vi "Canny Edge Detection Image.vi"() -> ()   [LabVIEW 2018]
doc: "Canny Edge Detection Image: This example is a Canny edge detection example, which is an image processing system that utilizes the Canny edge detection algorithm. Canny edge detection is a classic edge detection algorithm aimed at discovering strong edges in images and minimizing false detections and false edges as much as possible。"
uses:
  vi.lib/VIRobotics/opencv_yiku/Mat/Mat_8U/Mat_8U.lvclass
  D:/Program Files/Company/National Instruments/LabVIEW 2018(64bit)/vi.lib/addons/VIRobotics/opencv_yiku/Mat/Mat/Mat.lvclass
  vi.lib/VIRobotics/opencv_yiku/Mat/Create_Mat_8U.vi
  vi.lib/VIRobotics/opencv_yiku/opencv_yiku.lvlib
panel:
  out "edge":picture
  # "Overview: Demonstrates how to find edges with Canny Edge Detection\nRequirements: Windows.\nInstructions: \n1.Run the VI"
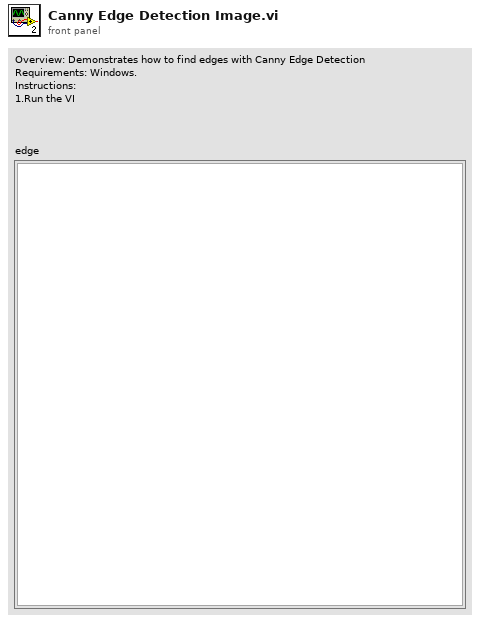
[diagram p1: front panel]
types:
  T1 = enum32{"COLOR_BGR2BGRA", "COLOR_BGRA2BGR", "COLOR_BGR2RGBA", "COLOR_RGBA2BGR", "COLOR_BGR2RGB", "COLOR_BGRA2RGBA", "COLOR_BGR2GRAY", "COLOR_RGB2GRAY", "COLOR_GRAY2BGR", "COLOR_GRAY2BGRA"}
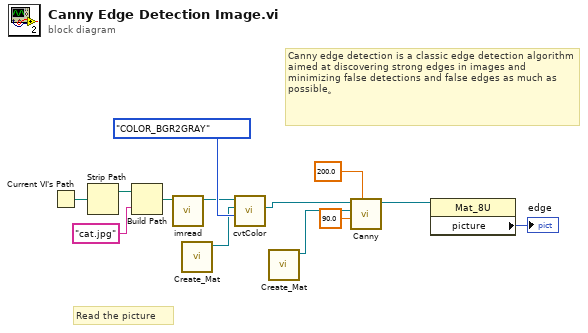
[diagram p0: block diagram]
diagram:
  # "Canny edge detection is a classic edge detection algorithm aimed at discovering strong edges in images and minimizing false detections and false edges as much as possible。"
  # "Read the picture"
  n1 = Current VI's Path() -> (path=w12:path)
  n2 = Strip Path(path=w12) -> (stripped path=w13:path)  [unwired: 1 out]
  n3 = Build Path(base path=w13, name or relative path="cat.jpg") -> (appended path=w10:path)
  n4 = call "imread.vi"("path"=w10) -> ("Mat out"=w8:refnum<class "Mat_8U.lvclass">)  [unwired: 9 in, 1 out]
  n5 = call-poly "Create_Mat.vi"() -> ("Mat_8U_out"=w2:refnum<class "Mat_8U.lvclass">)  [unwired: 10 in, 1 out]
  n6 = call "cvtColor.vi"("dstCn"=T1."COLOR_BGR2GRAY", "dst"=w2, "src"=w8) -> ("dst out"=w1:refnum<class "Mat_8U.lvclass">)  [unwired: 6 in, 2 out]
  n7 = call-poly "Create_Mat.vi"() -> ("Mat_8U_out"=w7:refnum<class "Mat_8U.lvclass">)  [unwired: 10 in, 1 out]
  n8 = call "Canny.vi"("threshold2"=200.0, "threshold1"=90.0, "dst in"=w7, "Mat in"=w1) -> ("dst out"=w4:refnum<class "Mat_8U.lvclass">)  [unwired: 6 in, 1 out]
  n9 = property class="Mat_8U"(reference=w4) -> ("picture"=→"edge":picture)  [unwired: 1 in, 2 out]
